vi "Firebase.vi"() -> ()   [LabVIEW 2022 SP3]
uses:
  <vilib>/httpClient/ClientHandle.ctl
  <vilib>/DAQmx/read.llb/DAQmx Read (Digital 1D Bool NChan 1Samp 1Line).vi
  <vilib>/DAQmx/read.llb/DAQmx Read (Analog 2D DBL NChan NSamp).vi
  <vilib>/Analysis/baseanly.llb/Mean (DBL).vi
  <vilib>/DAQmx/create/channels.llb/DAQmx Create Channel (AI-Temperature-Thermocouple).vi
  <vilib>/DAQmx/configure/timing.llb/DAQmx Timing (Sample Clock).vi
  <vilib>/DAQmx/miscellaneous.llb/DAQmx Fill In Error Info.vi
  <vilib>/httpClient/PUTBuffer.vi
  <vilib>/DAQmx/create/channels.llb/DAQmx Create Channel (DI-Digital Input).vi
  <vilib>/httpClient/LabVIEWHTTPClient.lvlib
  <vilib>/Analysis/NI_AALBase.lvlib
panel:
  out "Error":string
  out "test2":string
  out "temperature":string
  out "temperature_Raw_Data":string
  out "Start_Controller":string
  in  "Stop":dbl format="%#_13g"
  in  "Start":dbl format="%#_13g"
  in  "Stop":bool=TRUE
  in  "Start":bool=TRUE
  out "온도 데이터":string[][](array[string])
  out "온도 평균값":string[][](array[string])
  out "웹서버 전송 테스트":u32
  out "웹서버 전송 속도 test":u32
  out "URL":string
  out "루프 속도":u32
  out "body 2":string caption="값 출력"
  in  "데이타 쓰기":cluster{"0":string}
  out "data 2":bool[](array[boolean]) caption="DIO 입출력"
  in  "DIO 초기값":cluster{"line grouping":i32, "lines":tag}={"line grouping"=1, "lines"=""} {"line grouping" items=["각 라인에 하나의 채널", "모든 라인에 하나의 채널"]}
  in  "온도 초기값 설정":T1={"minimum value "=0.0, "maximum value "=100.0, "thermocouple type "=10072, "physical channels "=""} {"thermocouple type" items=["J"=10072, "K"=10073, "N"=10077, "R"=10082, "S"=10085, "T"=10086, "B"=10047, "E"=10055]}
  in  "샘플 속도":dbl=1000.0
  in  "데이터 값 출력":bool
  in  "데이터 값 전송":bool
  out "headers 2":string caption="연결확인 메세지 출력"
  in  "불리언":bool=TRUE
  # "웹서버 전송 프로젝트"
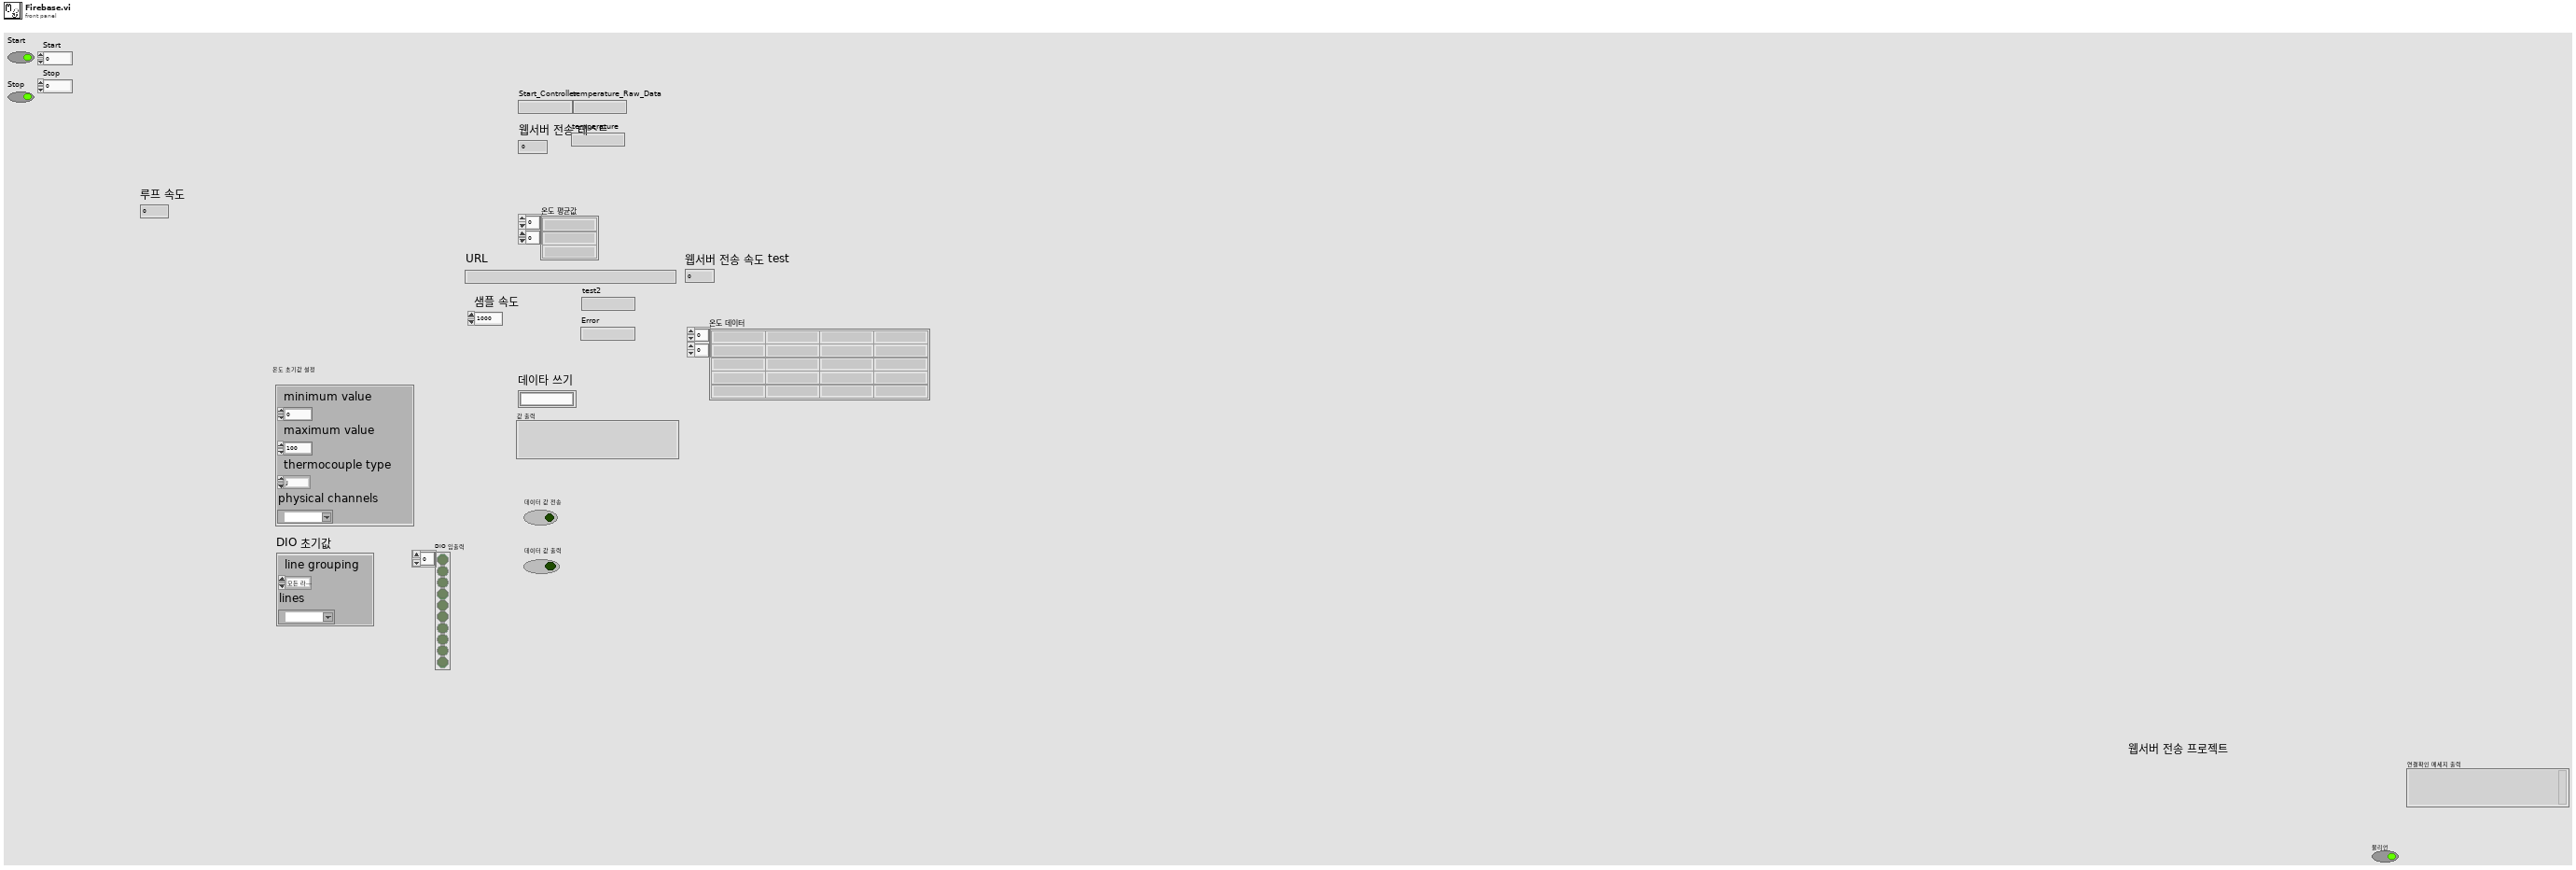
[diagram p1: front panel]
types:
  T1 = cluster{"minimum value ":dbl, "maximum value ":dbl, "thermocouple type ":i32, "physical channels ":tag}
  T2 = typedef "LabVIEWHTTPClient.lvlib/ClientHandle.ctl" = refnum<k1>
  T3 = typedef "웹서버 서버 컨트롤.ctl" = enum16{"초기화", "서버 전송", "서버 닫기"}
  T4 = typedef "웹서버 DAQ 제어 컨트롤.ctl" = enum16{"초기화", "측정대기", "측정 시작 ", "측정 종료"}
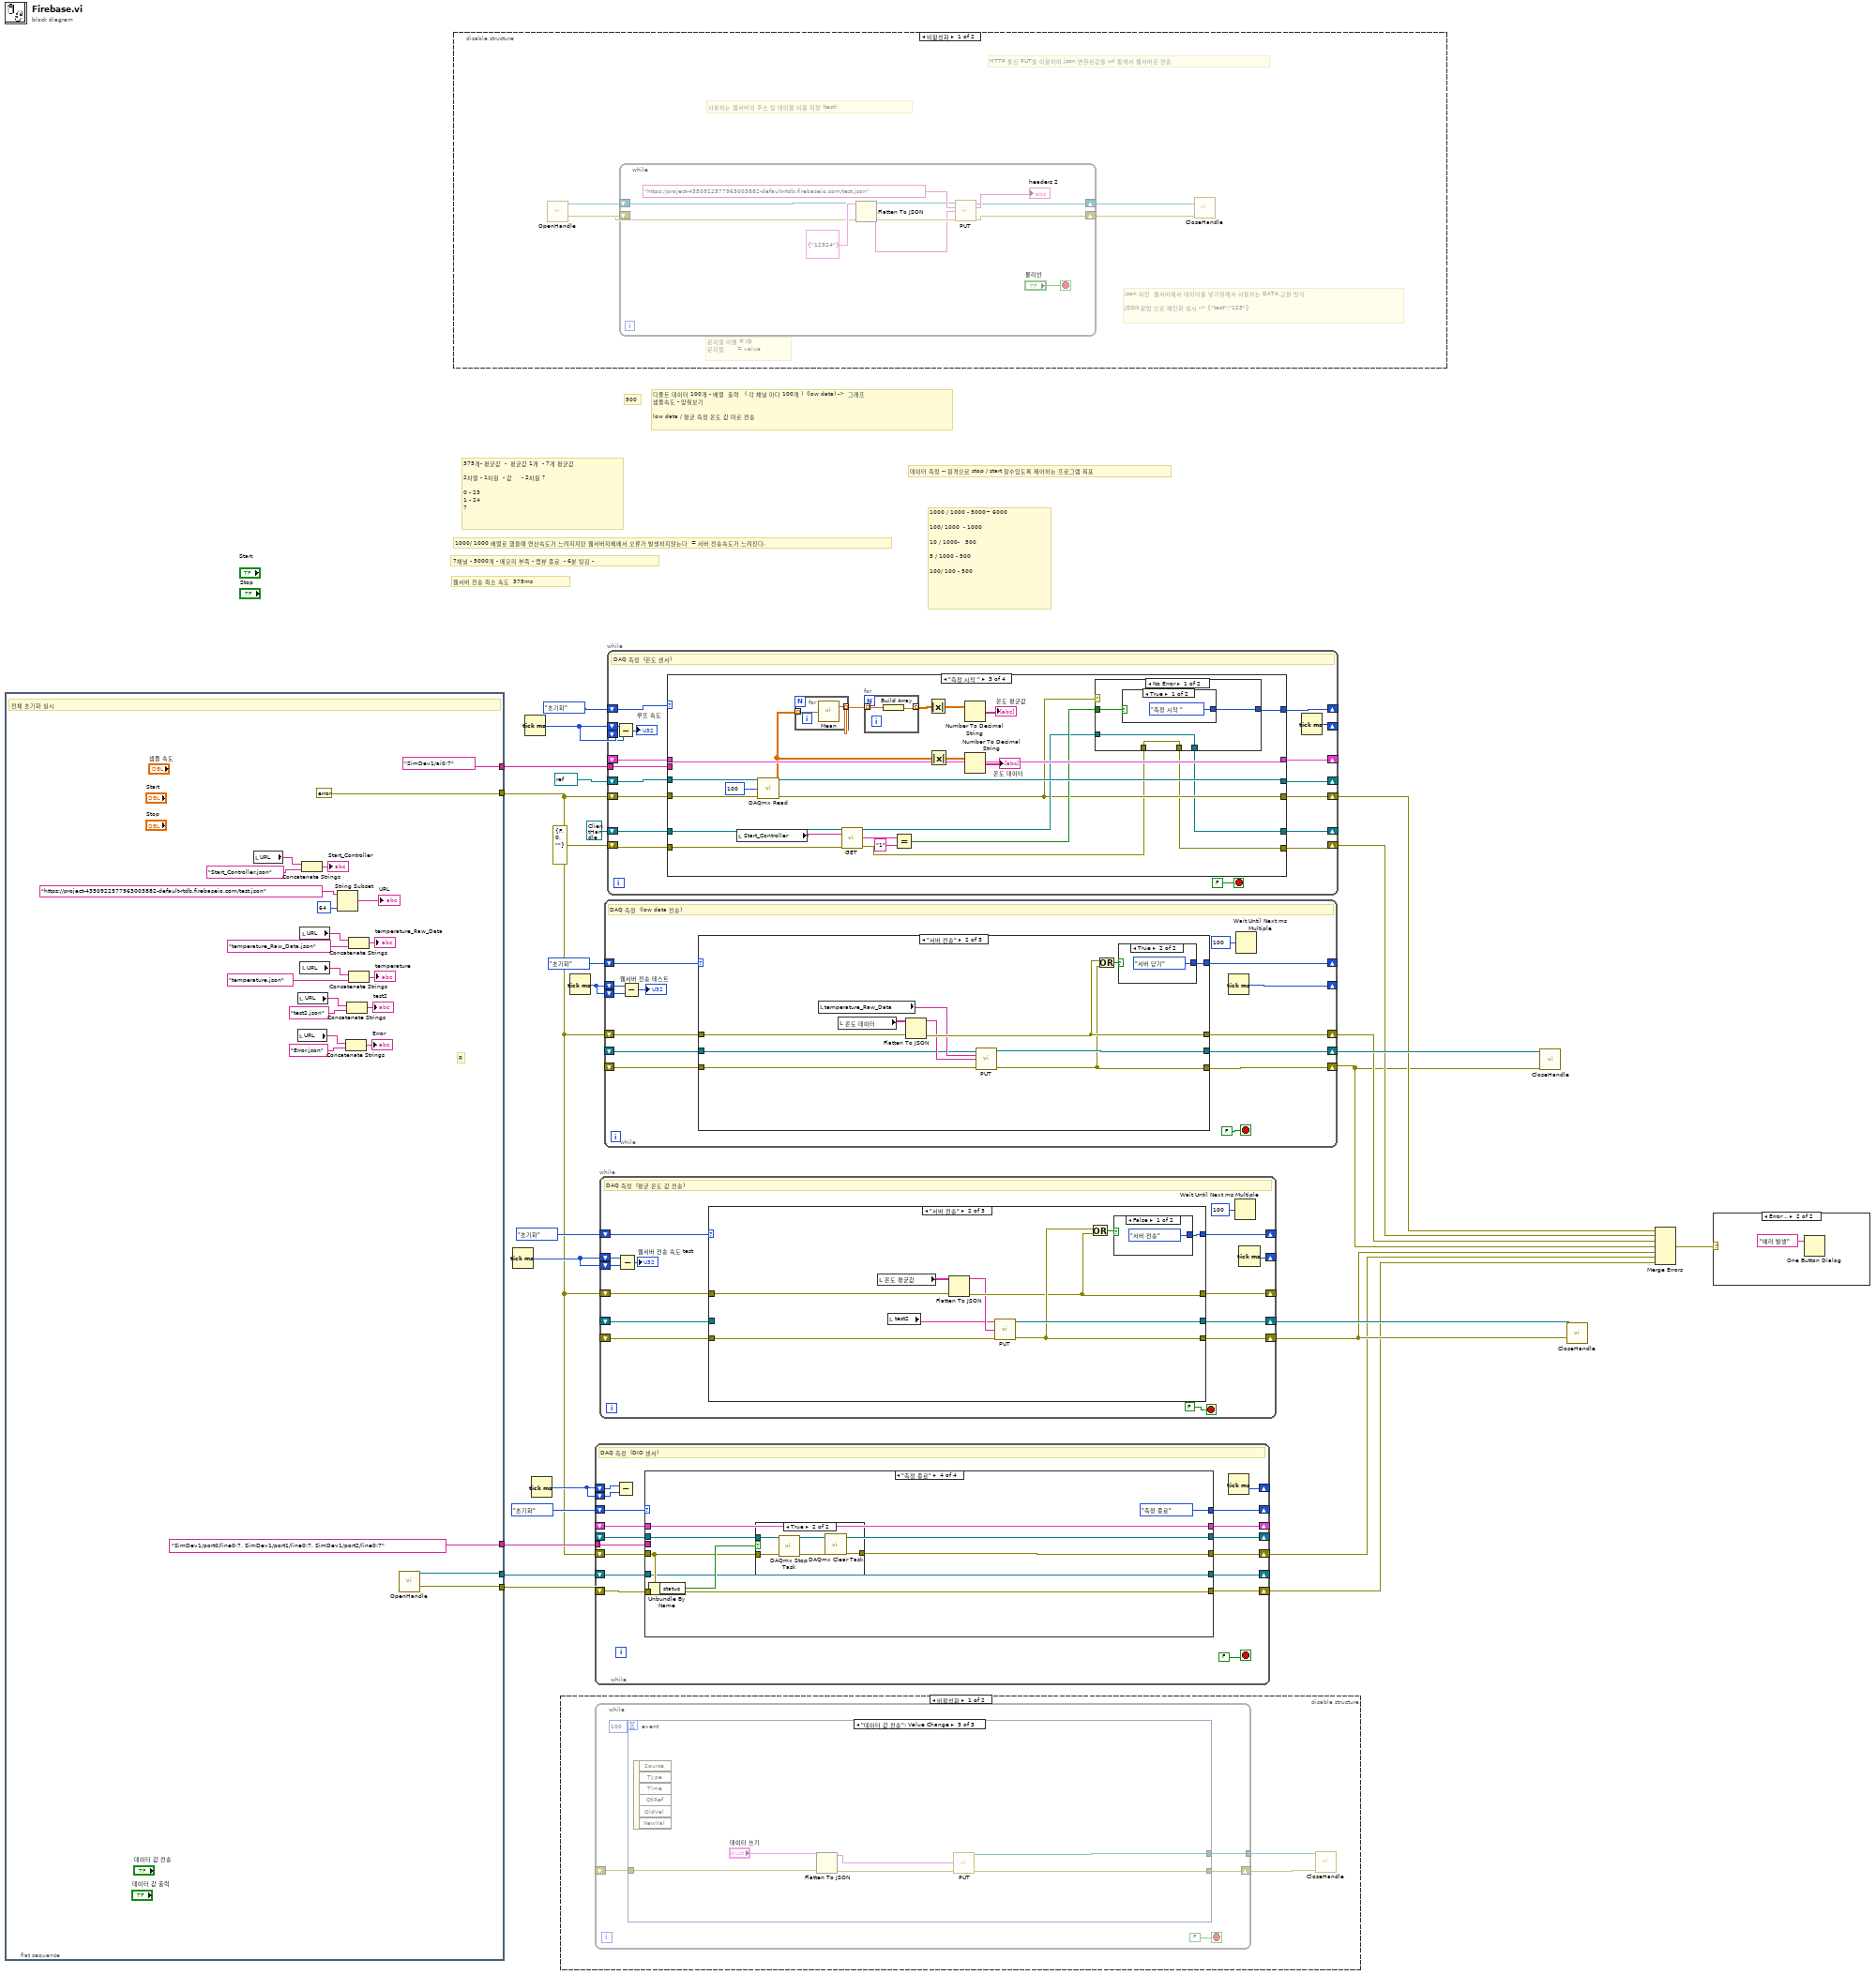
[diagram p0: block diagram]
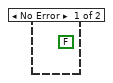
[diagram p2: hidden frame]
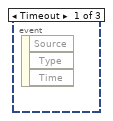
[diagram p3: hidden frame]
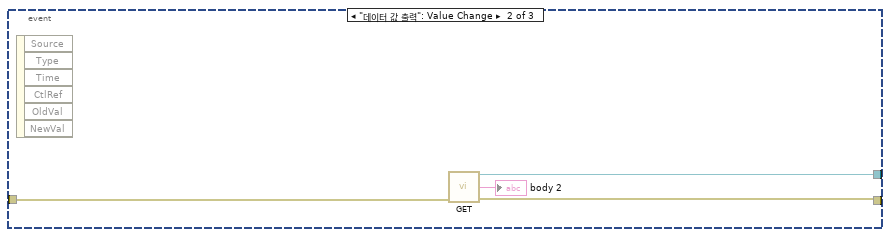
[diagram p4: hidden frame]
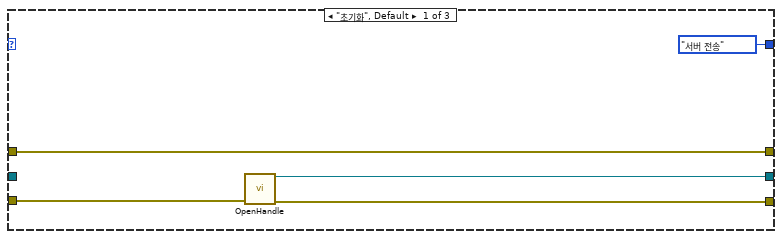
[diagram p6: hidden frame]
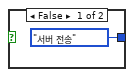
[diagram p7: hidden frame]
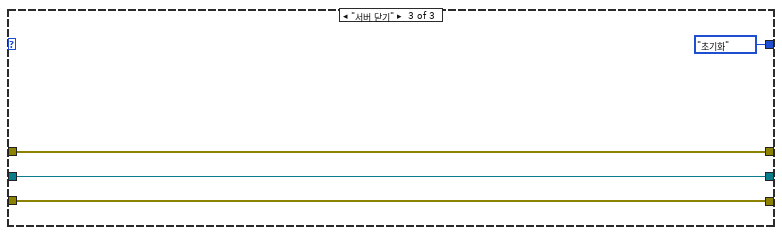
[diagram p8: hidden frame]
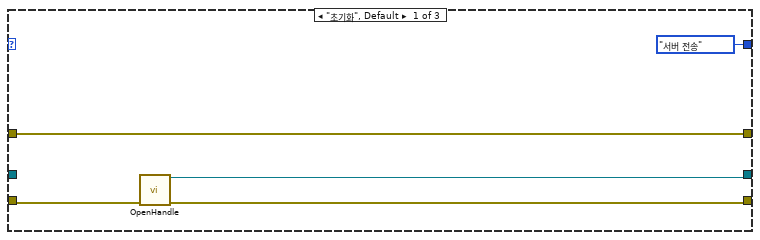
[diagram p9: hidden frame]
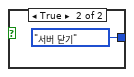
[diagram p10: hidden frame]
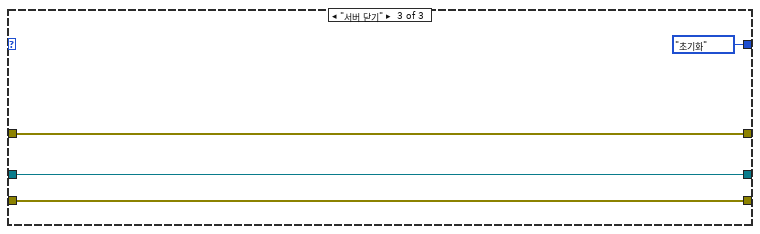
[diagram p11: hidden frame]
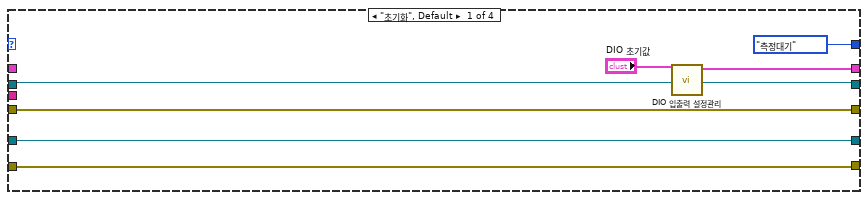
[diagram p12: hidden frame]
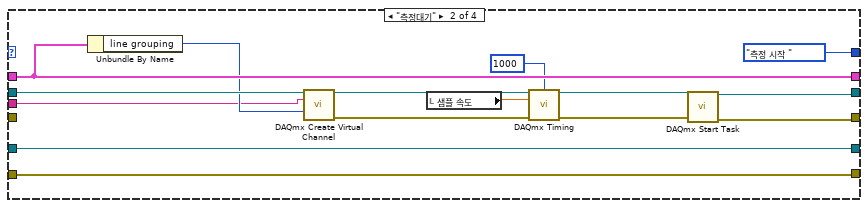
[diagram p13: hidden frame]
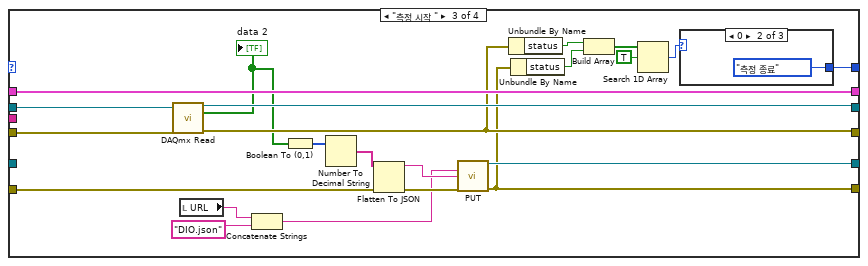
[diagram p14: hidden frame]
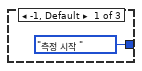
[diagram p15: hidden frame]
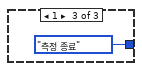
[diagram p16: hidden frame]
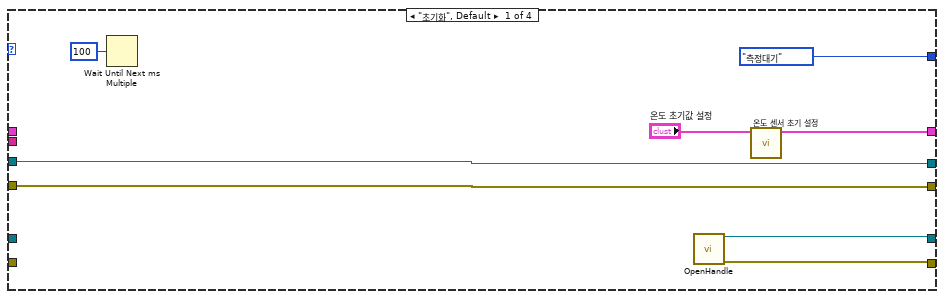
[diagram p18: hidden frame]
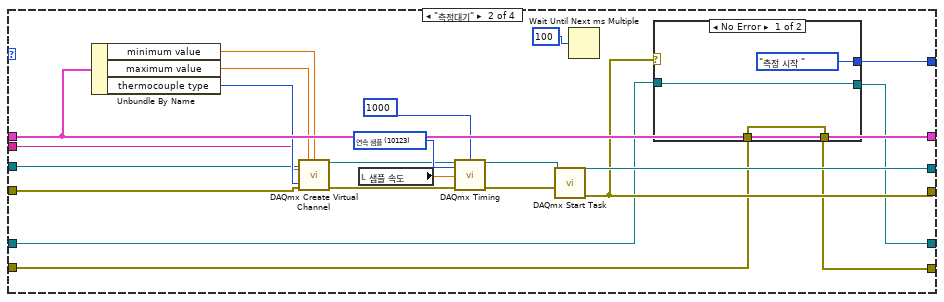
[diagram p19: hidden frame]
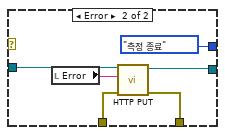
[diagram p20: hidden frame]
diagram:
  # "데이터 측정 -- 원격으로 stop / start 할수있도록 제어하는 프로그램 목표"
  # "1000 / 1000 - 5000~ 6000\n\n100/ 1000  - 1000\n\n10 / 1000-   500\n\n5 / 1000 - 500\n\n100/ 100 - 500"
  # "7채널 - 5000개 - 메모리 부족 - 랩뷰 종료  - 6분 팅김 -"
  # "1000/ 1000 배열로 했을때 연산속도가 느려지지만 웹서버자체에서 오류가 발생하지않는다  = 서버 전송속도가 느려진다."
  # "375개- 평균값  -  평균값 1개  - 7개 평균값 \n\n2차열 - 1차원  - 값     - 2차원 ?\n\n0 - 23\n1 - 24\n7"
  # "웹서버 전송 최소 속도  375ms"
  # "디폴트 데이터 100개 - 배열  출력   ( 각 채널 마다 100개 )  (low data) ->  그래프  \n샘플속도 - 맞춰보기 \n\nlow data / 평균 측정 온도 값 따로 전송"
  # "500"
  n1 = flat-sequence {
    tunnel: [errorcluster {"status"=FALSE, "code"=0, "source"=""} ("error in")] -> w10
    tunnel: [tag "SimDev1/port0/line0:7, SimDev1/port1/line0:7, SimDev1/port2/line0:7" ("lines")] -> w23
    tunnel: [w41] -> w18
    tunnel: [w40] -> w19
    tunnel: [tag "SimDev1/ai0:7" ("physical channels")] -> w1
    frame #0 {
      # "R"
      # "전체 초기화 실시"
      n2 = local read "URL"() -> (w43:string)
      n3 = local read "URL"() -> (w27:string)
      n4 = local read "URL"() -> (w32:string)
      n5 = local read "URL"() -> (w38:string)
      n6 = local read "URL"() -> (w33:string)
      n7 = Concatenate Strings(w43, "Start_Controller.json" ("문자열")) -> (→"Start_Controller":string)
      n8 = String Subset(string="https://project-4350922577963003882-default-rtdb.firebaseio.com/test.json" ("url"), length (rest)=64 ("길이(나머지)")) -> (substring=→"URL":string)  [unwired: 1 in]
      n9 = Concatenate Strings(w27, "Error.json" ("문자열")) -> (→"Error":string)
      n10 = Concatenate Strings(w32, "test2.json" ("문자열")) -> (→"test2":string)
      n11 = Concatenate Strings(w38, "temperature_Raw_Data.json") -> (→"temperature_Raw_Data":string)
      n12 = Concatenate Strings(w33, "temperature.json") -> (→"temperature":string)
      n13 = call <vilib>:"OpenHandle.vi"() -> ("client handle out"=w41:T2, "error out"=w40:errorcluster)  [unwired: 14 in]
    }
  }
  n14 = disable-structure shown="비활성화" {
    frame Disabled {
      # "문자열 라벨 = ID \n문자열       = value"
      # "HTTP 통신 PUT을 이용하여 json 변환된값을 url 통해서 웹서버로 전송"
      # "사용하는 웹서버의 주소 및 테이블 이름 지정 (test)"
      # "json 이란  웹서버에서 데이터를 넣기위해서 사용하는 DATA 교환 방식\n\nJSON 문법 으로 패턴화 실시 -> {\"test\":\"123\"}"
      n15 = call <vilib>:"OpenHandle.vi"() -> ("client handle out"=w53:T2, "error out"=w52:errorcluster)  [unwired: 14 in]
      n16 = while {
        shift-right: [w56] -> w50
        shift-left: w53 -> [w54]
        shift-right: [w57] -> w51
        shift-left: w52 -> [w62]
        stop <- "불리언" stop-if-true
        n17 = Flatten To JSON(anything=cluster{"값":string} {"값"="12324"} ("임의의 데이터"), error in (no error)=w62) -> (JSON string=w55:string, 11:w58:errorcluster)  [unwired: 1 in]
        n18 = call-poly <vilib>:"PUT.vi"("client handle"=w54, "url"="https://project-4350922577963003882-default-rtdb.firebaseio.com/test.json", "buffer"=w55, "error in (no error)"=w58) -> ("client handle out"=w56:T2, "headers"=→"headers 2":string, "body"=w59:string, "error out"=w57:errorcluster)  [unwired: 8 in]
      }
      n19 = call <vilib>:"CloseHandle.vi"("client handle"=w50, "error in (no error)"=w51) -> ()  [unwired: 13 in, 1 out]
    }
    frame Enabled {
    }
  }
  n20 = Tick Count (ms)() -> (millisecond timer value=w20:u32)
  n21 = Tick Count (ms)() -> (millisecond timer value=w22:u32)
  n22 = Tick Count (ms)() -> (millisecond timer value=w21:u32)
  n23 = disable-structure shown="비활성화" {
    frame Disabled {
      n24 = while {
        shift-right: [w69] -> w65
        shift-left: _ -> [w68]
        tunnel: [w67] -> w66
        stop <- FALSE stop-if-true
        n25 = event shown="[2] \"데이터 값 전송\": Value Change" {
          selector: _ -> [_ _ _]
          dyn-events: _ -> [_ _ _]
          timeout: 100 -> [_ _ _]
          tunnel: w68 -> [_ w74 w81]
          tunnel: [_ w72 w77] -> w69
          tunnel: [_ w73 w76] -> w67
          event Timeout {
            n26 = event-data() -> ()  [unwired: 1 in, 3 out]
          }
          event "데이터 값 출력": Value Change {
            n27 = event-data() -> ()  [unwired: 1 in, 6 out]
            n28 = call <vilib>:"GET.vi"("error in (no error)"=w74) -> ("client handle out"=w73:T2, "body"=→"body 2":string, "error out"=w72:errorcluster)  [unwired: 11 in, 1 out]
          }
          event "데이터 값 전송": Value Change {
            n29 = event-data() -> ()  [unwired: 1 in, 6 out]
            n30 = Flatten To JSON(anything="데이타 쓰기", error in (no error)=w81) -> (JSON string=w79:string, 11:w78:errorcluster)  [unwired: 1 in]
            n31 = call-poly <vilib>:"PUT.vi"("buffer"=w79, "error in (no error)"=w78) -> ("client handle out"=w76:T2, "error out"=w77:errorcluster)  [unwired: 10 in, 2 out]
          }
        }
      }
      n32 = call <vilib>:"CloseHandle.vi"("client handle"=w66, "error in (no error)"=w65) -> ()  [unwired: 13 in, 1 out]
    }
    frame Enabled {
    }
  }
  n33 = Tick Count (ms)() -> (millisecond timer value=w16:u32)
  n34 = while {
    shift-right: [w96] -> _
    shift-left: 웹서버_DAQ_제어_컨트롤."초기화" -> [w97]
    shift-right: [w95] -> _
    shift-left: _ -> [w94]
    shift-right: [w92] -> _
    shift-left: _ -> [w93]
    shift-right: [w91] -> w4
    shift-left: w10 -> [w90]
    tunnel: w23 -> [w89]
    shift-right: [w87] -> w3
    shift-left: w19 -> [w86]
    shift-right: [w85] -> _
    shift-left: w21 -> [w84]
    shift-left: w21 -> [w83]
    shift-right: [w88] -> _
    shift-left: w18 -> [w82]
    stop <- FALSE stop-if-true
    # "DAQ 측정  (DIO 센서)"
    n35 = Subtract(x=w84, y=w83) -> ()  [unwired: 1 out]
    n36 = case shown="\"측정 종료\"" w97 {
      tunnel: [웹서버_DAQ_제어_컨트롤."측정대기" 웹서버_DAQ_제어_컨트롤."측정 시작 " w138 웹서버_DAQ_제어_컨트롤."측정 종료"] -> w96
      tunnel: [w104 w119 w142 w153] -> w95
      tunnel: w94 -> [_ w119 w142 w153]
      tunnel: w93 -> [w103 w118 w141 w150]
      tunnel: [w103 w110 w139 w150] -> w92
      tunnel: [w102 w109 w137 w148] -> w91
      tunnel: w90 -> [w102 _ w140 w149]
      tunnel: w89 -> [_ w116 _ _]
      tunnel: w86 -> [w100 w108 w131 w147]
      tunnel: [w99 w107 w136 w146] -> w88
      tunnel: [w100 w108 w129 w147] -> w87
      tunnel: w82 -> [w99 w107 _ w146]
      frame "초기화", Default {
        n37 = call "DIO 입출력 설정관리.vi"("클러스터"="DIO 초기값") -> ("출력 클러스터"=w104:cluster{"line grouping":i32, "lines":tag})  [unwired: 10 in]
      }
      frame "측정대기" {
        n38 = Unbundle By Name(w119) -> ("line grouping"=w117:i32)
        n39 = call-poly <vilib>:"DAQmx Create Virtual Channel.vi"("task in"=w118, "lines"=w116, "line grouping"=w117) -> ("task out"=w115:refnum<k21>, "error out"=w114:errorcluster)  [unwired: 11 in]
        n40 = local read "샘플 속도"() -> (w106:dbl)
        n41 = call-poly <vilib>:"DAQmx Timing.vi"("task/channels in"=w115, "samples per channel"=1000, "rate"=w106, "error in"=w114) -> ("task out"=w112:refnum<k21>, "error out"=w111:errorcluster)  [unwired: 10 in]
        n42 = call <vilib>:"DAQmx Start Task.vi"("task/channels in"=w112, "error in"=w111) -> ("task out"=w110:refnum<k21>, "error out"=w109:errorcluster)  [unwired: 12 in]
      }
      frame "측정 시작 " {
        n43 = call-poly <vilib>:"DAQmx Read.vi"("task/channels in"=w141, "error in"=w140) -> ("task out"=w139:refnum<k21>, "data"=w134:bool[], "error out"=w137:errorcluster)  [unwired: 11 in]
        "data 2" <- w134
        n44 = local read "URL"() -> (w122:string)
        n45 = Concatenate Strings(w122, "DIO.json" ("문자열")) -> (w121:string)
        n46 = Boolean To (0,1)(Boolean=w134) -> (0, 1=w135:i16[])
        n47 = Number To Decimal String(number=w135) -> (decimal integer string=w133:string[])  [unwired: 1 in]
        n48 = Flatten To JSON(anything=w133, error in (no error)=w131) -> (JSON string=w132:string, 11:w130:errorcluster)  [unwired: 1 in]
        n49 = call-poly <vilib>:"PUT.vi"("url"=w121, "buffer"=w132, "error in (no error)"=w130) -> ("client handle out"=w136:T2, "error out"=w129:errorcluster)  [unwired: 9 in, 2 out]
        n50 = Unbundle By Name(w137) -> ("status"=w128:bool)
        n51 = Unbundle By Name(w129) -> ("status"=w127:bool)
        n52 = Build Array(w128, w127) -> (w126:bool[])
        n53 = Search 1D Array(1D array=w126, element=TRUE ("원소")) -> (index of element=w124:i32)  [unwired: 1 in]
        n54 = case shown="0" w124 {
          tunnel: [웹서버_DAQ_제어_컨트롤."측정 시작 " 웹서버_DAQ_제어_컨트롤."측정 종료" 웹서버_DAQ_제어_컨트롤."측정 종료"] -> w138
          frame -1, Default {
          }
          frame 0 {
          }
          frame 1 {
          }
        }
      }
      frame "측정 종료" {
        n55 = Unbundle By Name(w149) -> ("status"=w151:bool)
        n56 = case shown="True" w151 {
          tunnel: w149 -> [w154 w157]
          tunnel: [w154 w156] -> w148
          tunnel: w150 -> [_ w155]
          frame False {
          }
          frame True {
            n57 = call <vilib>:"DAQmx Stop Task.vi"("task/channels in"=w155, "error in"=w157) -> ("task out"=w159:refnum<k21>, "error out"=w158:errorcluster)  [unwired: 12 in]
            n58 = call <vilib>:"DAQmx Clear Task.vi"("task in"=w159, "error in"=w158) -> ("error out"=w156:errorcluster)  [unwired: 13 in]
          }
        }
      }
    }
    n59 = Tick Count (ms)() -> (millisecond timer value=w85:u32)
  }
  n60 = while {
    shift-right: [w172] -> w12
    shift-left: _ -> [w170]
    shift-right: [w171] -> w5
    shift-left: _ -> [w169]
    shift-right: [w168] -> _
    shift-left: w20 -> [w167]
    shift-left: w20 -> [w166]
    shift-right: [w163] -> _
    shift-left: 웹서버_서버_컨트롤."초기화" -> [w164]
    shift-right: [w162] -> _
    shift-left: w10 -> [w161]
    stop <- FALSE stop-if-true
    # "DAQ 측정  (평균 온도 값 전송)"
    n61 = Subtract(x=w167, y=w166) -> (x-y=→"웹서버 전송 속도 test":u32)
    n62 = case shown="\"서버 전송\"" w164 {
      tunnel: [w175 w188 w192] -> w172
      tunnel: [w174 w186 w191] -> w171
      tunnel: w170 -> [_ _ w192]
      tunnel: w169 -> [w177 w180 w191]
      tunnel: [웹서버_서버_컨트롤."서버 전송" w187 웹서버_서버_컨트롤."초기화"] -> w163
      tunnel: [w176 w185 w193] -> w162
      tunnel: w161 -> [w176 w181 w193]
      frame "초기화", Default {
        n63 = call <vilib>:"OpenHandle.vi"("error in (no error)"=w177) -> ("client handle out"=w175:T2, "error out"=w174:errorcluster)  [unwired: 13 in]
      }
      frame "서버 전송" {
        n64 = local read "온도 평균값"() -> (w182:string[][])
        n65 = local read "test2"() -> (w179:string)
        n66 = Flatten To JSON(anything=w182, error in (no error)=w181) -> (JSON string=w183:string, 11:w185:errorcluster)  [unwired: 1 in]
        n67 = call-poly <vilib>:"PUT.vi"("url"=w179, "buffer"=w183, "error in (no error)"=w180) -> ("client handle out"=w188:T2, "error out"=w186:errorcluster)  [unwired: 9 in, 2 out]
        n68 = Or(x=w186, y=w185) -> (x .or. y?=w184:bool)
        n69 = case shown="False" w184 {
          tunnel: [웹서버_서버_컨트롤."서버 전송" 웹서버_서버_컨트롤."서버 닫기"] -> w187
          frame False {
          }
          frame True {
          }
        }
      }
      frame "서버 닫기" {
      }
    }
    n70 = Wait Until Next ms Multiple(millisecond multiple=u32 100 ("ms 배수")) -> ()  [unwired: 1 out]
    n71 = Tick Count (ms)() -> (millisecond timer value=w168:u32)
  }
  n72 = while {
    shift-right: [w207] -> w13
    shift-left: _ -> [w205]
    shift-right: [w206] -> w6
    shift-left: _ -> [w204]
    shift-right: [w203] -> _
    shift-left: w16 -> [w199]
    shift-left: w16 -> [w198]
    shift-right: [w201] -> _
    shift-left: 웹서버_서버_컨트롤."초기화" -> [w202]
    shift-right: [w200] -> w7
    shift-left: w10 -> [w196]
    stop <- FALSE stop-if-true
    # "DAQ 측정  (low data 전송)"
    n73 = Subtract(x=w199, y=w198) -> (x-y=→"웹서버 전송 테스트":u32)
    n74 = case shown="\"서버 전송\"" w202 {
      tunnel: [w211 w224 w228] -> w207
      tunnel: [w210 w220 w227] -> w206
      tunnel: w205 -> [_ w215 w228]
      tunnel: w204 -> [w212 w214 w227]
      tunnel: [웹서버_서버_컨트롤."서버 전송" w223 웹서버_서버_컨트롤."초기화"] -> w201
      tunnel: [w209 w221 w229] -> w200
      tunnel: w196 -> [w209 w222 w229]
      frame "초기화", Default {
        n75 = call <vilib>:"OpenHandle.vi"("error in (no error)"=w212) -> ("client handle out"=w211:T2, "error out"=w210:errorcluster)  [unwired: 13 in]
      }
      frame "서버 전송" {
        n76 = local read "temperature_Raw_Data"() -> (w216:string)
        n77 = local read "온도 데이터"() -> (w217:string[][])
        n78 = Flatten To JSON(anything=w217, error in (no error)=w222) -> (JSON string=w218:string, 11:w221:errorcluster)  [unwired: 1 in]
        n79 = call-poly <vilib>:"PUT.vi"("client handle"=w215, "url"=w216, "buffer"=w218, "error in (no error)"=w214) -> ("client handle out"=w224:T2, "error out"=w220:errorcluster)  [unwired: 8 in, 2 out]
        n80 = Or(x=w221, y=w220) -> (x .or. y?=w219:bool)
        n81 = case shown="True" w219 {
          tunnel: [웹서버_서버_컨트롤."서버 전송" 웹서버_서버_컨트롤."서버 닫기"] -> w223
          frame False {
          }
          frame True {
          }
        }
      }
      frame "서버 닫기" {
      }
    }
    n82 = Tick Count (ms)() -> (millisecond timer value=w203:u32)
    n83 = Wait Until Next ms Multiple(millisecond multiple=u32 100 ("ms 배수")) -> ()  [unwired: 1 out]
  }
  n84 = while {
    shift-right: [w246] -> _
    shift-left: 웹서버_DAQ_제어_컨트롤."초기화" -> [w247]
    shift-right: [w245] -> _
    shift-left: _ -> [w244]
    shift-right: [w242] -> _
    shift-left: refnum<k21> refnum ("task in") -> [w243]
    tunnel: w1 -> [w241]
    shift-right: [w240] -> _
    shift-left: w22 -> [w239]
    shift-left: w22 -> [w238]
    shift-right: [w236] -> _
    shift-left: T2 refnum ("client handle out") -> [w234]
    shift-right: [w235] -> w8
    shift-left: errorcluster {"status"=FALSE, "code"=0, "source"=""} ("error out") -> [w233]
    shift-right: [w231] -> w9
    shift-left: w10 -> [w232]
    stop <- FALSE stop-if-true
    # "DAQ 측정  (온도 센서)"
    n85 = Subtract(x=w239, y=w238) -> (x-y=→"루프 속도":u32)
    n86 = case shown="\"측정 시작 \"" w247 {
      tunnel: [웹서버_DAQ_제어_컨트롤."측정대기" w261 w310 웹서버_DAQ_제어_컨트롤."초기화"] -> w246
      tunnel: [w255 w278 w311 w343] -> w245
      tunnel: w244 -> [_ w278 w311 w343]
      tunnel: w243 -> [w254 w274 w309 w341]
      tunnel: [w254 w267 w308 w339] -> w242
      tunnel: w241 -> [_ w266 _ _]
      tunnel: [w250 w259 w288 w331] -> w236
      tunnel: [w249 w257 w289 w338] -> w235
      tunnel: w234 -> [_ w260 w298 w329]
      tunnel: w233 -> [_ w258 w299 w328]
      tunnel: [w251 w262 w291 w336] -> w231
      tunnel: w232 -> [w251 w263 w297 w335]
      frame "초기화", Default {
        n87 = Wait Until Next ms Multiple(millisecond multiple=u32 100 ("ms 배수")) -> ()  [unwired: 1 out]
        n88 = call <vilib>:"OpenHandle.vi"() -> ("client handle out"=w250:T2, "error out"=w249:errorcluster)  [unwired: 14 in]
        n89 = call "온도 센서 초기 설정.vi"("클러스터"="온도 초기값 설정") -> ("출력 클러스터"=w255:T1)  [unwired: 10 in]
      }
      frame "측정대기" {
        w273 = 10123 items=["유한 샘플"=10178, "연속 샘플"=10123, "하드웨어 타이밍에 의한 단일 포인트"=12522] ("sample mode")
        n90 = Unbundle By Name(w278) -> ("minimum value"=w277:dbl, "maximum value"=w276:dbl, "thermocouple type"=w275:i32)
        n91 = call-poly <vilib>:"DAQmx Create Virtual Channel.vi"("task in"=w274, "maximum value"=w276, "minimum value"=w277, "physical channels"=w266, "error in"=w263, "thermocouple type"=w275) -> ("task out"=w271:refnum<k21>, "error out"=w270:errorcluster)  [unwired: 8 in]
        n92 = local read "샘플 속도"() -> (w264:dbl)
        n93 = call-poly <vilib>:"DAQmx Timing.vi"("task/channels in"=w271, "sample mode"=w273, "samples per channel"=1000, "rate"=w264, "error in"=w270) -> ("task out"=w269:refnum<k21>, "error out"=w268:errorcluster)  [unwired: 9 in]
        n94 = call <vilib>:"DAQmx Start Task.vi"("task/channels in"=w269, "error in"=w268) -> ("task out"=w267:refnum<k21>, "error out"=w262:errorcluster)  [unwired: 12 in]
        n95 = Wait Until Next ms Multiple(millisecond multiple=u32 100 ("ms 배수")) -> ()  [unwired: 1 out]
        n96 = case shown="No Error" w262 {
          tunnel: [웹서버_DAQ_제어_컨트롤."측정 시작 " 웹서버_DAQ_제어_컨트롤."측정 종료"] -> w261
          tunnel: w260 -> [w279 w286]
          tunnel: [w279 w285] -> w259
          tunnel: w258 -> [w280 w282]
          tunnel: [w280 w283] -> w257
          frame No Error {
          }
          frame Error {
            n97 = local read "Error"() -> (w284:string)
            n98 = call "HTTP PUT.vi"("error in (no error)"=w282, "url"=w284, "참조 번호 입력"=w286) -> ("에러 출력"=w283:errorcluster, "참조 번호 출력"=w285:T2)  [unwired: 7 in]
          }
        }
      }
      frame "측정 시작 " {
        n99 = local read "Start_Controller"() -> (w303:string)
        n100 = call-poly <vilib>:"DAQmx Read.vi"("task/channels in"=w309, "number of samples per channel"=100, "error in"=w297) -> ("task out"=w308:refnum<k21>, "data"=w293:dbl[][], "error out"=w291:errorcluster)  [unwired: 10 in]
        n101 = for {
          tunnel: w293 -> [w327] mode=indexing
          tunnel: [w326] -> w306 mode=indexing
          n102 = call-poly <vilib>:"Mean.vi"("X"=w327) -> ("mean"=w326:dbl)  [unwired: 1 out]
        }
        n103 = call <vilib>:"GET.vi"("client handle"=w298, "url"=w303, "error in (no error)"=w299) -> ("client handle out"=w292:T2, "body"=w301:string, "error out"=w290:errorcluster)  [unwired: 9 in, 1 out]
        n104 = for {
          tunnel: w306 -> [w324] mode=indexing
          tunnel: [w325] -> w296 mode=indexing
          n105 = Build Array(w324) -> (w325:dbl[])
        }
        n106 = Equal?(x=w301, y="1") -> (x = y?=w300:bool)
        n107 = Absolute Value(x=w296) -> (abs(x)=w295:dbl[][])
        n108 = Absolute Value(x=w293) -> (abs(x)=w294:dbl[][])
        n109 = Number To Decimal String(number=w295) -> (decimal integer string=→"온도 평균값":string[][])  [unwired: 1 in]
        n110 = Number To Decimal String(number=w294) -> (decimal integer string=→"온도 데이터":string[][])  [unwired: 1 in]
        n111 = case shown="No Error" w291 {
          tunnel: [w315 웹서버_DAQ_제어_컨트롤."측정 종료"] -> w310
          tunnel: w300 -> [w314 _]
          tunnel: w292 -> [w312 w322]
          tunnel: w290 -> [w313 w320]
          tunnel: [w313 w319] -> w289
          tunnel: [w312 w318] -> w288
          frame No Error {
            n112 = case shown="True" w314 {
              tunnel: [웹서버_DAQ_제어_컨트롤."측정 시작 " 웹서버_DAQ_제어_컨트롤."측정 종료"] -> w315
              frame True {
              }
              frame False {
              }
            }
          }
          frame Error {
            n113 = local read "Error"() -> (w321:string)
            n114 = call "HTTP PUT.vi"("error in (no error)"=w320, "url"=w321, "참조 번호 입력"=w322) -> ("에러 출력"=w319:errorcluster, "참조 번호 출력"=w318:T2)  [unwired: 7 in]
          }
        }
      }
      frame "측정 종료" {
        n115 = call <vilib>:"DAQmx Stop Task.vi"("task/channels in"=w341, "error in"=w335) -> ("task out"=w339:refnum<k21>, "error out"=w337:errorcluster)  [unwired: 12 in]
        n116 = call <vilib>:"DAQmx Clear Task.vi"("task in"=w339, "error in"=w337) -> ("error out"=w336:errorcluster)  [unwired: 13 in]
        n117 = Wait Until Next ms Multiple(millisecond multiple=u32 100 ("ms 배수")) -> ()  [unwired: 1 out]
        n118 = local read "Start_Controller"() -> (w334:string)
        n119 = Flatten To JSON(anything=cluster{string} {"0"} ("임의의 데이터")) -> (JSON string=w333:string)  [unwired: 2 in, 1 out]
        n120 = call-poly <vilib>:"PUT.vi"("client handle"=w329, "url"=w334, "buffer"=w333, "error in (no error)"=w328) -> ("client handle out"=w331:T2, "error out"=w330:errorcluster)  [unwired: 8 in, 2 out]
        n121 = call <vilib>:"CloseHandle.vi"("client handle"=w331, "error in (no error)"=w330) -> ("error out"=w338:errorcluster)  [unwired: 13 in]
      }
    }
    n122 = Tick Count (ms)() -> (millisecond timer value=w240:u32)
  }
  n123 = call <vilib>:"CloseHandle.vi"("client handle"=w13, "error in (no error)"=w6) -> ()  [unwired: 13 in, 1 out]
  n124 = call <vilib>:"CloseHandle.vi"("client handle"=w12, "error in (no error)"=w5) -> ()  [unwired: 13 in, 1 out]
  n125 = Merge Errors(w9, w8, w7, w6, w5, w4, w3) -> (w2:errorcluster)
  n126 = case shown="Error .." w2 {
    frame No Error {
      (unwired) FALSE ("종료? (참)")
    }
    frame Error {
      n127 = One Button Dialog(message="에러 발생" ("메시지")) -> ()  [unwired: 1 in, 1 out]
    }
  }
